vi "Variant to Display Metadata.vi"(8 "error in":errorcluster, 11 "value":variant) -> (0 "error out":errorcluster, 1 "display metadata":T1, 2 "found?":bool, 3 "value out":variant)   [LabVIEW 2020, in "Value.lvlib"]
uses:
  Value.lvlib
  Display Metadata.ctl
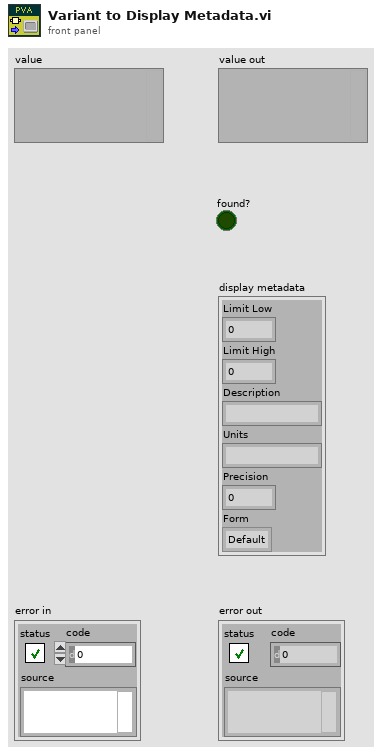
[diagram p1: front panel]
types:
  T1 = typedef "Value.lvlib/Display Metadata.ctl" = cluster{"Limit Low":dbl, "Limit High":dbl, "Description":string, "Units":string, "Precision":i32, "Form":enum32{"Default", "String", "Binary", "Decimal", "Hex", "Exponential", "Engineering"}}
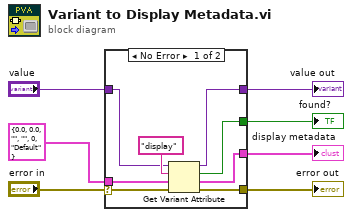
[diagram p0: block diagram]
diagram:
  n1 = case shown="No Error" "error in" {
    selector: "error in" -> [w14 w17]
    tunnel: [w11 w17] -> w7
    tunnel: "value" -> [w13 w16]
    tunnel: [w12 w16] -> w4
    tunnel: [w9 _] -> w2
    tunnel: T1 {"Limit Low"=0.0, "Limit High"=0.0, "Description"="", "Units"="", "Precision"=0, "Form"=enum."Default"} ("Display") -> [w10 _]
    tunnel: [w8 _] -> w1
    frame No Error {
      n2 = Get Variant Attribute(Variant=w13, name="display", default value (empty Variant)=w10, error in=w14) -> (duplicate Variant=w12:variant, found=w8:bool, value=w9:T1, error out=w11:errorcluster)
    }
    frame Error {
    }
  }
  "error out" <- w7
  "value out" <- w4
  "display metadata" <- w2
  "found?" <- w1
